vi "GetTheTypeAndValue.vi"(8 "error in (no error)":errorcluster, 11 "Data Cluster":T1) -> (0 "error out":errorcluster, 3 "DataType and Value":cluster{"Type":string, "Value":variant})   [LabVIEW 2017]
uses:
  Ctrl/User Input Cluster.ctl
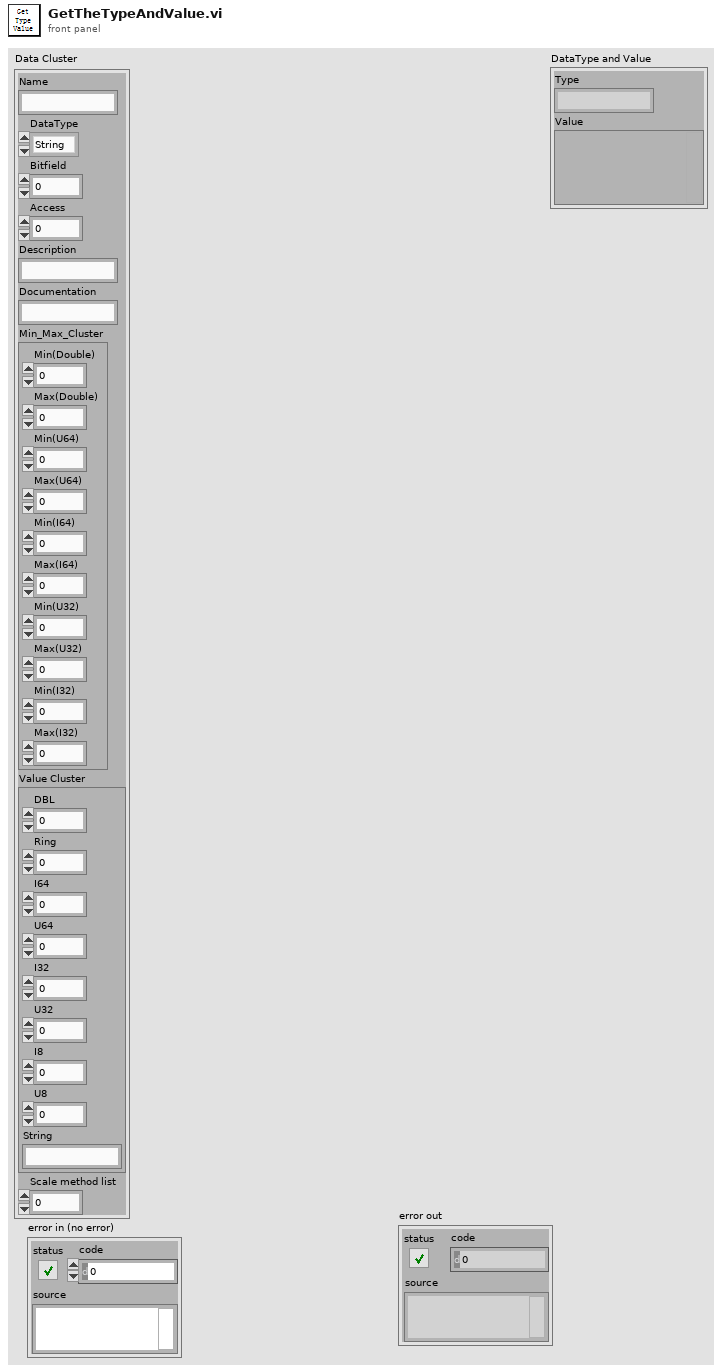
[diagram p1: front panel]
types:
  T1 = typedef "User Input Cluster.ctl" = cluster{"Name":string, "DataType":enum16{"String", "Double", "U64", "I64", "U32", "I32", "Bool"}, "Bitfield":u16, "Access":u16, "Description":string, "Documentation":string, "Min_Max_Cluster":cluster{"Min(Double)":dbl, "Max(Double)":dbl, "Min(U64)":u64, "Max(U64)":u64, "Min(I64)":i64, "Max(I64)":i64, "Min(U32)":u32, "Max(U32)":u32, "Min(I32)":i32, "Max(I32)":i32}, "Value Cluster":cluster{"DBL":dbl, "Ring":u16, "I64":i64, "U64":u64, "I32":i32, "U32":u32, "I8":i8, "U8":u8, "String":string}, "Scale method list":u16}
  T2 = enum16{"String", "Double", "U64", "I64", "U32", "I32", "Bool"}
  T3 = cluster{"DBL":dbl, "Ring":u16, "I64":i64, "U64":u64, "I32":i32, "U32":u32, "I8":i8, "U8":u8, "String":string}
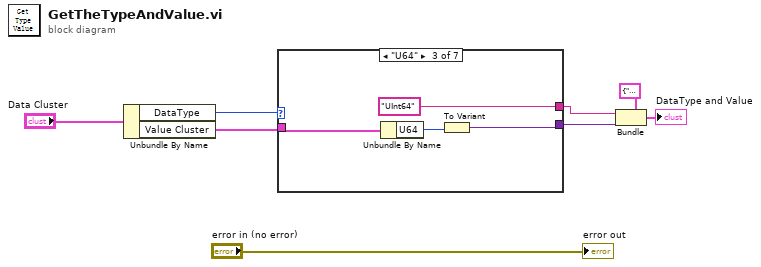
[diagram p0: block diagram]
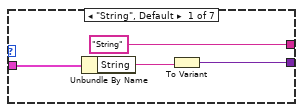
[diagram p2: hidden frame]
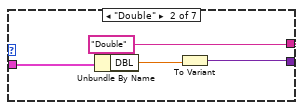
[diagram p3: hidden frame]
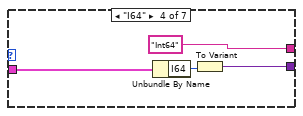
[diagram p4: hidden frame]
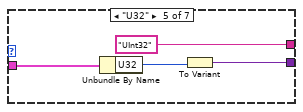
[diagram p5: hidden frame]
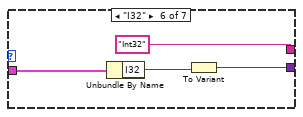
[diagram p6: hidden frame]
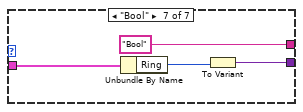
[diagram p7: hidden frame]
diagram:
  n1 = Unbundle By Name("Data Cluster") -> ("DataType"=w7:T2, "Value Cluster"=w6:T3)
  n2 = case shown="\"U64\"" w7 {
    tunnel: w6 -> [w10 w16 w17 w21 w25 w29 w35]
    tunnel: ["String" "Double" "UInt64" "Int64" "UInt32" "Int32" "Bool"] -> w4
    tunnel: [w11 w13 w19 w23 w27 w31 w34] -> w3
    frame "String", Default {
      n3 = Unbundle By Name(w10) -> ("String"=w9:string)
      n4 = To Variant(anything=w9) -> (Variant=w11:variant)
    }
    frame "Double" {
      n5 = Unbundle By Name(w16) -> ("DBL"=w15:dbl)
      n6 = To Variant(anything=w15) -> (Variant=w13:variant)
    }
    frame "U64" {
      n7 = Unbundle By Name(w17) -> ("U64"=w20:u64)
      n8 = To Variant(anything=w20) -> (Variant=w19:variant)
    }
    frame "I64" {
      n9 = Unbundle By Name(w21) -> ("I64"=w24:i64)
      n10 = To Variant(anything=w24) -> (Variant=w23:variant)
    }
    frame "U32" {
      n11 = Unbundle By Name(w25) -> ("U32"=w28:u32)
      n12 = To Variant(anything=w28) -> (Variant=w27:variant)
    }
    frame "I32" {
      n13 = Unbundle By Name(w29) -> ("I32"=w32:i32)
      n14 = To Variant(anything=w32) -> (Variant=w31:variant)
    }
    frame "Bool" {
      n15 = Unbundle By Name(w35) -> ("Ring"=w36:u16)
      n16 = To Variant(anything=w36) -> (Variant=w34:variant)
    }
  }
  n17 = Bundle(cluster=cluster{"Type":string, "Value":variant} {"Type"="", "Value"=variant}, "Type"=w4, "Value"=w3) -> (→"DataType and Value":cluster{"Type":string, "Value":variant})
  "error out" <- "error in (no error)"
